vi "256-bit CHDR Header.vi"(6 "timestamp (0)":u64, 7 "reset":bool, 9 "ready for output":bool, 10 "aurora frame length":u16, 11 "header parameters":T1) -> (3 "chdr header":bool[](array[boolean]))   [LabVIEW 2023, in "CHDR Support.lvlib"]
doc: "Generates a CHDR header based on the profided parameters. Includes counters for the <b>Sequence Number</b> and <b>End of Vector</b> and <b>End of Burst<b/> signals."
uses:
  CHDR Support.lvlib
  <instrlib>/_niInstr/Basic Elements/v1/FPGA/Private/Count Up U16.vi
  <instrlib>/_niInstr/Basic Elements/v1/FPGA/niInstr Basic Elements v1 FPGA.lvlib
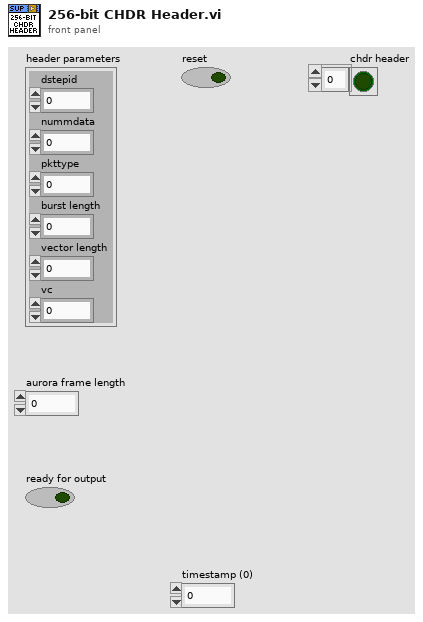
[diagram p1: front panel]
types:
  T1 = cluster{"dstepid":u16, "nummdata":fxp<+,5,5>, "pkttype":fxp<+,3,3>, "burst length":u16, "vector length":u16, "vc":fxp<+,6,6>}
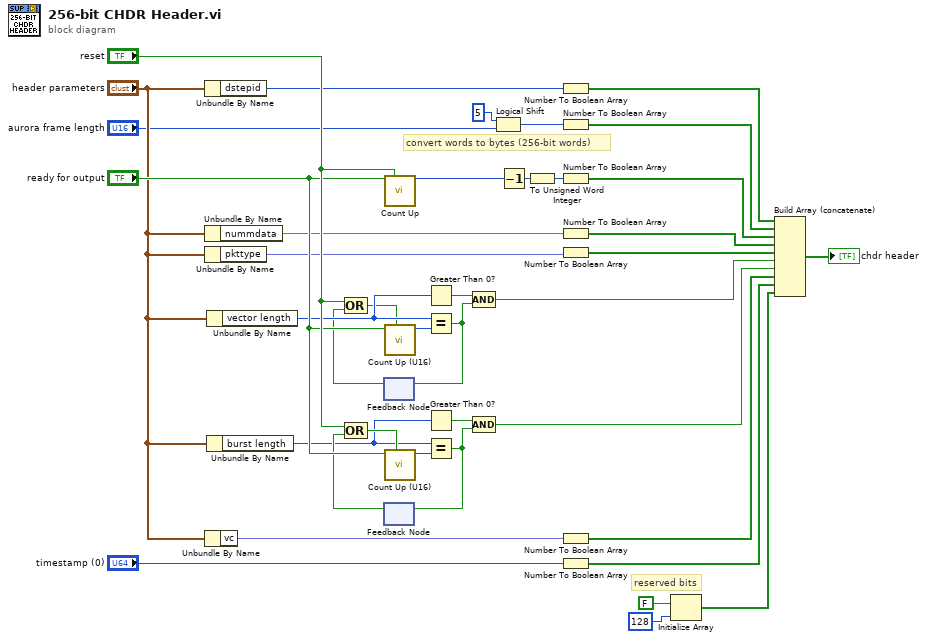
[diagram p0: block diagram]
diagram:
  # "reserved bits"
  # "convert words to bytes (256-bit words)"
  n1 = Unbundle By Name("header parameters") -> ("dstepid"=w16:u16)
  n2 = Unbundle By Name("header parameters") -> ("nummdata"=w17:fxp<+,5,5>)
  n3 = Unbundle By Name("header parameters") -> ("pkttype"=w18:fxp<+,3,3>)
  n4 = Unbundle By Name("header parameters") -> ("vc"=w19:fxp<+,6,6>)
  n5 = Unbundle By Name("header parameters") -> ("vector length"=w33:u16)
  n6 = Unbundle By Name("header parameters") -> ("burst length"=w22:u16)
  n7 = feedback #1() -> (w28:bool)  [unwired: 1 in]
  n8 = Compound Arithmetic op=OR("reset", w28) -> (w29:bool)
  n9 = feedback #2() -> (w26:bool)  [unwired: 1 in]
  n10 = Compound Arithmetic op=OR("reset", w26) -> (w25:bool)
  n11 = call-poly <instrlib>:"Count Up.vi"("increment"="ready for output", "reset"="reset") -> ("count out"=w35:u16)  [unwired: 13 in]
  n12 = call "Count Up (U16).vi"("reset"=w29, "increment"="ready for output") -> ("count out"=w32:u16)  [unwired: 9 in]
  n13 = call "Count Up (U16).vi"("reset"=w25, "increment"="ready for output") -> ("count out"=w20:u16)  [unwired: 9 in]
  n14 = Greater Than 0?(x=w33) -> (x > 0?=w31:bool)
  n15 = Equal?(x=w33, y=w32) -> (x = y?=w30:bool)
  n16 = feedback-in #1(w30) -> ()
  n17 = Greater Than 0?(x=w22) -> (x > 0?=w23:bool)
  n18 = Equal?(x=w22, y=w20) -> (x = y?=w24:bool)
  n19 = feedback-in #2(w24) -> ()
  n20 = Compound Arithmetic op=AND(w31, w30) -> (w34:bool)
  n21 = Compound Arithmetic op=AND(w23, w24) -> (w27:bool)
  n22 = Logical Shift(y=i16 5, x="aurora frame length") -> (x << y=w7:u16)
  n23 = Decrement(x=w35) -> (x-1=w38:u16)
  n24 = To Unsigned Word Integer(number=w38) -> (unsigned 16bit integer=w8:u16)
  n25 = Number To Boolean Array(number=w16) -> (Boolean array=w9:bool[])
  n26 = Number To Boolean Array(number=w7) -> (Boolean array=w10:bool[])
  n27 = Number To Boolean Array(number=w8) -> (Boolean array=w11:bool[])
  n28 = Number To Boolean Array(number=w17) -> (Boolean array=w12:bool[])
  n29 = Number To Boolean Array(number=w18) -> (Boolean array=w13:bool[])
  n30 = Number To Boolean Array(number=w19) -> (Boolean array=w14:bool[])
  n31 = Number To Boolean Array(number="timestamp (0)") -> (Boolean array=w15:bool[])
  n32 = Initialize Array(FALSE, 128 ("dimension size")) -> (w2:bool[])
  n33 = Build Array (concatenate)(w9, w10, w11, w12, w13, w34, w27, w14, w15, w2) -> (→"chdr header":bool[])
